vi "F.vi"(1 "Promien krzywizny południka [v]":ext, 2 "fi[rad]":ext) -> (0 "D":ext)   [LabVIEW 2012, in "Biblioteka moduł map v3.lvlib" / "Konwersja wsp.lvlib" / "UTM.lvlib" / "Konwersja na UTM.lvlib"]
doc: "Współczynnik wzoru na konwersję na UTM."
uses:
  Konwersja na UTM.lvlib
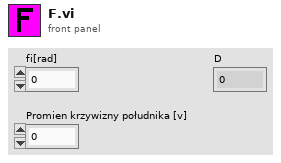
[diagram p1: front panel]
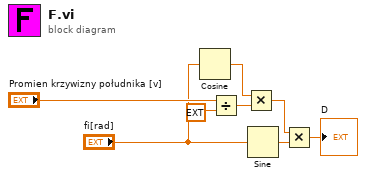
[diagram p0: block diagram]
diagram:
  n1 = Cosine(x="fi[rad]") -> (cos(x)=w3:ext)
  n2 = Divide(x="Promien krzywizny południka [v]", y=ext 2.0) -> (x/y=w6:ext)
  n3 = Multiply(x=w3, y=w6) -> (x*y=w7:ext)
  n4 = Sine(x="fi[rad]") -> (sin(x)=w1:ext)
  n5 = Multiply(x=w7, y=w1) -> (x*y=→"D":ext)
